vi "VIUsingSubVI.vi"() -> ()   [LabVIEW 2018]
panel:
  out "?":dbl(knob) scale=0.0..10.0
  in  "Knob":dbl(knob) scale=0.0..1000.0
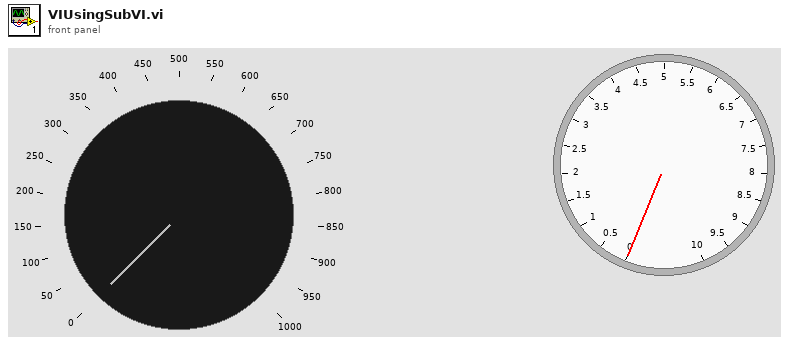
[diagram p1: front panel]
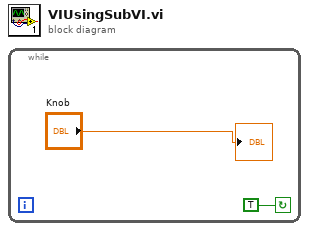
[diagram p0: block diagram]
diagram:
  n1 = while {
    stop <- TRUE continue-if-true
    "?" <- "Knob"
  }
